vi "WPI_CameraERRFailedComm.vi"() -> (0 "error out":errorcluster)   [LabVIEW 2017]
doc: "This software is licensed. Open the labview\\readme\\WPI Robotics Library Open Source License.txt file for more information."
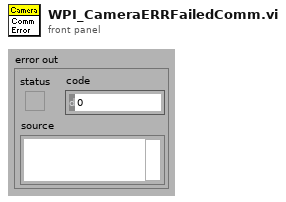
[diagram p1: front panel]
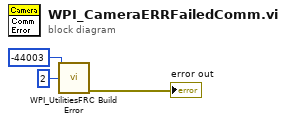
[diagram p0: block diagram]
diagram:
  n1 = call <vilib>:"WPI_UtilitiesFRC Build Error.vi"("error code"=-44003 ("code"), "chain levels to remove (1)"=2) -> ("error out"=→"error out":errorcluster)  [unwired: 3 in, 10 out]
